vi "ReadStandStatus.vi"(8 "error in":errorcluster, 10 "milliseconds to wait":u32=50, 11 "VISA resource name":refnum<visa-resource-name>) -> (0 "error out":errorcluster, 2 "Status":string, 3 "VISA resource name out":refnum<visa-resource-name>)   [LabVIEW 2019, in "Mark 10 TSTM-DC.lvlib"]
uses:
  Mark 10 TSTM-DC.lvlib
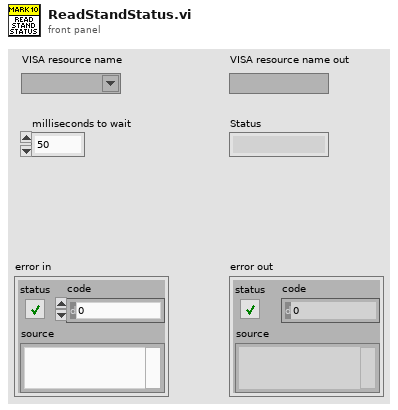
[diagram p1: front panel]
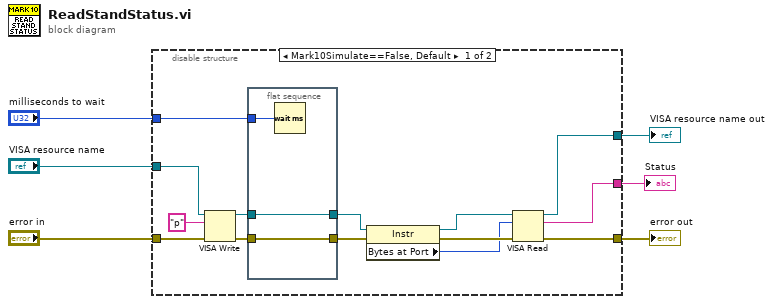
[diagram p0: block diagram]
diagram:
  n1 = disable-structure shown="Mark10Simulate==False, Default" {
    disable-tunnel: [w20 w25] -> w6
    disable-tunnel: "VISA resource name" -> [w19 w25]
    disable-tunnel: "error in" -> [w18 w24]
    disable-tunnel: [w17 w24] -> w3
    disable-tunnel: "milliseconds to wait" -> [w16 _]
    disable-tunnel: [w15 _] -> w1
    frame condition #0 (active) {
      n2 = VISA Write(VISA resource name=w19, write buffer="p" ("String to Write"), error in (no error)=w18) -> (VISA resource name out=w10:refnum<visa-resource-name>, error out=w9:errorcluster)  [unwired: 1 out]
      n3 = flat-sequence {
        tunnel: [w23] -> w11
        tunnel: w10 -> [w23]
        tunnel: w9 -> [w22]
        tunnel: [w22] -> w8
        tunnel: w16 -> [w21]
        frame #0 {
          n4 = Wait (ms)(milliseconds to wait=w21) -> ()  [unwired: 1 out]
        }
      }
      n5 = property class="Instr"(reference=w11, error in=w8) -> (reference out=w12:refnum<visa-resource-name>, error out=w13:errorcluster, "Bytes at Port"=w7:u32)
      n6 = VISA Read(VISA resource name=w12, byte count=w7, error in (no error)=w13) -> (VISA resource name out=w20:refnum<visa-resource-name>, read buffer=w15:string, error out=w17:errorcluster)  [unwired: 1 out]
    }
    frame condition #1 {
    }
  }
  "error out" <- w3
  "VISA resource name out" <- w6
  "Status" <- w1
